vi "Send Command.vi"(8 "error in":errorcluster, 9 "Value":variant, 10 "Command":string, 11 "DAQ970 in":refnum<class "DAQ970.lvclass">) -> (0 "error out":errorcluster, 3 "DAQ970 out":refnum<class "DAQ970.lvclass">)   [LabVIEW 2019, in "DAQ970.lvlib" / "DAQ970.lvclass"]
uses:
  Library/DAQ970.lvclass
  C:/Users/Public/Documents/Development/builds/Engine/Engine.lvlibp/Project/Engine.lvclass
  DAQ970 Messages/Toggle By Name Msg/Toggle By Name Msg.lvclass/Toggle By Name Msg.ctl
  builds/Engine/Engine.lvlibp/Accessors/Read Self Q.vi
  builds/Engine/Actor Framework.lvlibp/1abvi3w/vi.lib/ActorFramework/Message Enqueuer/Enqueue.vi
  builds/Engine/Actor Framework.lvlibp/1abvi3w/vi.lib/ActorFramework/Message Enqueuer/Message Enqueuer.lvclass
  DAQ970 Messages/Toggle By Name Msg/Toggle By Name Msg.lvclass
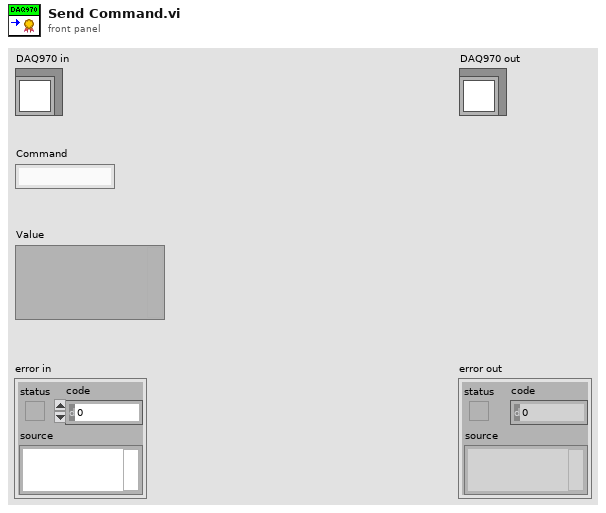
[diagram p1: front panel]
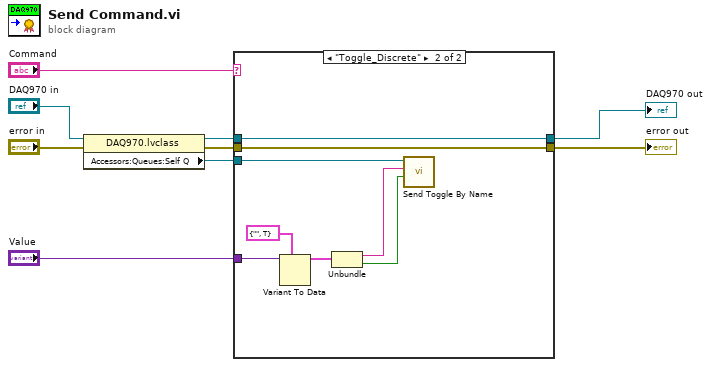
[diagram p0: block diagram]
diagram:
  n1 = property class="DAQ970.lvclass"(reference="DAQ970 in", error in="error in") -> (reference out=w5:refnum<class "DAQ970.lvclass">, error out=w3:errorcluster, "Accessors:Queues:Self Q"=w1:refnum<class "Message Enqueuer.lvclass">)
  n2 = case shown="\"Toggle_Discrete\"" "Command" {
    tunnel: "Value" -> [_ w17]
    tunnel: w5 -> [w11 w19]
    tunnel: [w11 w19] -> w4
    tunnel: [w10 w18] -> w2
    tunnel: w3 -> [w10 w18]
    tunnel: w1 -> [_ w14]
    frame "False", Default {
    }
    frame "Toggle_Discrete" {
      n3 = Variant To Data(type=cluster{"Name":string, "State":bool} {"Name"="", "State"=TRUE}, Variant=w17) -> (data=w16:cluster{"Name":string, "State":bool})  [unwired: 1 in, 1 out]
      n4 = Unbundle(w16) -> ("Name"=w13:string, "State"=w12:bool)
      n5 = call "Send Toggle By Name.vi"("State"=w12, "Name"=w13, "Message Enqueuer"=w14) -> ()  [unwired: 7 in, 2 out]
    }
  }
  "error out" <- w2
  "DAQ970 out" <- w4
